vi "NextState.vi"(0 "object in":refnum<class "PrimaryAttackerRole.lvclass">, 2 "Robot in":refnum<class "Robot.lvclass">, 4 "GameRef":refnum<data-value>, 5 "error in (no error)":errorcluster) -> (14 "object out":refnum<class "PrimaryAttackerRole.lvclass">, 16 "Robot out":refnum<class "Robot.lvclass">, 19 "error out":errorcluster)   [LabVIEW 2023, in "PrimaryAttackerRole.lvclass"]
uses:
  PrimaryAttackerRole.lvclass
  C:/Users/ebert/Documents/codes/SSL/repo/SSL_AI/NewSTP/NewRoles/Role_v2_class/Role_v2.lvclass
  Robot_class/Robot.lvclass
  Game_class/Game.lvclass
  PrimaryAttackerRole_states.ctl
  Robot_class/tactics.ctl
  Game_class/Game.lvclass/Game.ctl
  Field_class/Field.lvclass/Field.ctl
  Robot_class/Robot.lvclass/Robot.ctl
  Game_class/Read FieldRef.vi
  Field_class/Read enemyGoalPosition.vi
  Robot_class/Write tactic.vi
  Field_class/Field.lvclass
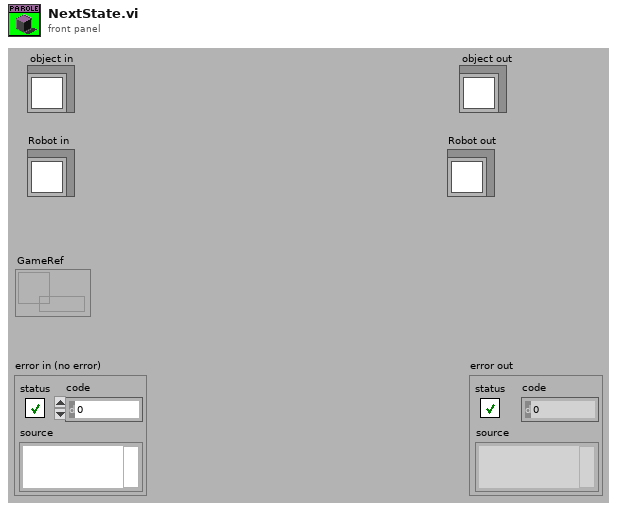
[diagram p1: front panel]
types:
  T1 = typedef "PrimaryAttackerRole.lvclass/PrimaryAttackerRole_states.ctl" = enum16{"Intercept", "PrepareShot", "Shoot", "Pass"}
  T2 = typedef "tactics.ctl" = enum16{"GoToBallPlacementPosition", "PlaceBall", "GoToBallPlacement", "5Robots", "BallPlacementEnemy", "ReceivePassInFuturePoint", "Roller", "PrepareRollToPassRollerGoTo", "PrepareRollToPassReceiverGoTo", "WaitRoll", "PositionToRoll", "PenaltyAttacker", "PassObserver", "PenaltyDefense", "TableReceiverTactic", "Test", "DefendGoal", "Marker", "FollowAttacker", "DefendArea", "Shoot", "AttackerAimGoal", "AttackerBallOutOfField", "AttackerBlock", "AttackerStop", "Duelist", "Halt", "ZigZag", "GoTo", "Timeout", "KickToBestRobot", "KickToPassReceiver", "PositionToReceivePass", "WaitPass", "Position", "Intercept", "PrepareShot", "Pass"}
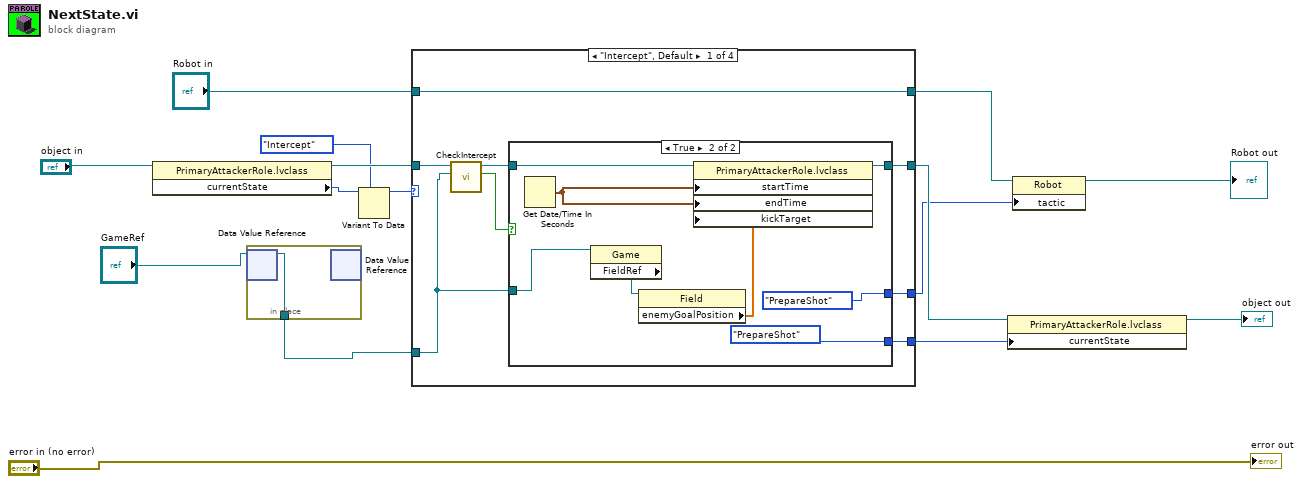
[diagram p0: block diagram]
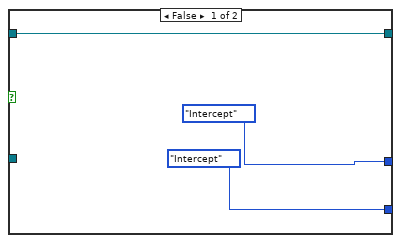
[diagram p2: hidden frame]
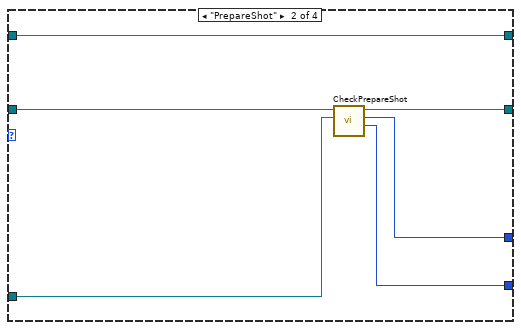
[diagram p3: hidden frame]
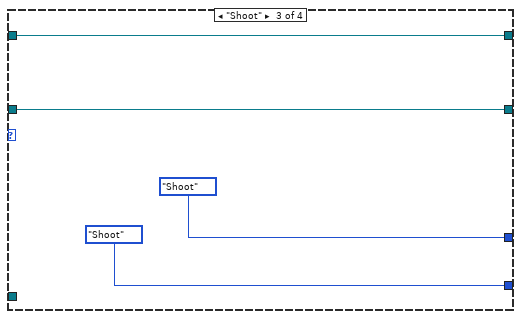
[diagram p4: hidden frame]
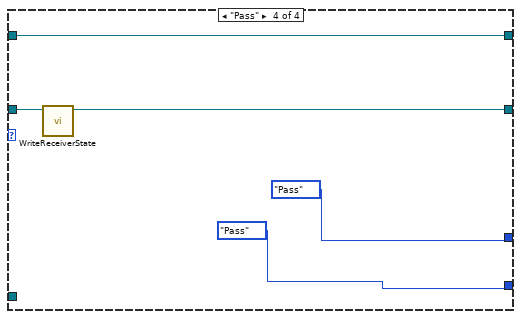
[diagram p5: hidden frame]
diagram:
  n1 = property class="PrimaryAttackerRole.lvclass"(reference="object in") -> (reference out=w13:refnum<class "PrimaryAttackerRole.lvclass">, "currentState"=w7:u8)  [unwired: 1 in, 1 out]
  n2 = in-place {
    in-place-border: [w16] -> w1
    n3 = in-place-dvr #1("GameRef") -> (w16:refnum<class "Game.lvclass">)  [unwired: 1 out]
    n4 = in-place-dvr #1() -> ()  [unwired: 1 in, 2 out]
  }
  n5 = Variant To Data(type=PrimaryAttackerRole_states."Intercept" ("Enum"), Variant=w7) -> (data=w5:T1)  [unwired: 1 in, 1 out]
  n6 = case shown="\"Intercept\", Default" w5 {
    tunnel: [w22 w38 PrimaryAttackerRole_states."Shoot" ("Enum") PrimaryAttackerRole_states."Pass" ("Enum")] -> w3
    tunnel: w1 -> [w17 w37 _ _]
    tunnel: w13 -> [w24 w41 w43 w48]
    tunnel: [w19 w40 w43 w47] -> w14
    tunnel: [w21 w39 tactics."Shoot" ("tactic") tactics."Pass" ("tactic")] -> w4
    tunnel: "Robot in" -> [w18 w36 w42 w46]
    tunnel: [w18 w36 w42 w46] -> w8
    frame "Intercept", Default {
      n7 = call-dynamic "CheckIntercept.vi"("Game"=w17, "object in"=w24) -> ("intercepted"=w23:bool, "object out"=w20:refnum<class "PrimaryAttackerRole.lvclass">)  [unwired: 7 in, 1 out]
      n8 = case shown="True" w23 {
        tunnel: [PrimaryAttackerRole_states."Intercept" ("Enum") PrimaryAttackerRole_states."PrepareShot" ("Enum")] -> w22
        tunnel: [tactics."Intercept" ("tactic") tactics."PrepareShot" ("tactic")] -> w21
        tunnel: w20 -> [w25 w33]
        tunnel: [w25 w32] -> w19
        tunnel: w17 -> [_ w28]
        frame False {
        }
        frame True {
          n9 = Get Date/Time In Seconds() -> (seconds since 1Jan1904=w31:timestamp)
          n10 = property class="Game"(reference=w28) -> ("FieldRef"=w30:refnum<class "Field.lvclass">)  [unwired: 1 in, 2 out]
          n11 = property class="Field"(reference=w30) -> ("enemyGoalPosition"=w29:dbl[])  [unwired: 1 in, 2 out]
          n12 = property class="PrimaryAttackerRole.lvclass"(reference=w33, "startTime"=w31, "endTime"=w31, "kickTarget"=w29) -> (reference out=w32:refnum<class "PrimaryAttackerRole.lvclass">)  [unwired: 1 in, 1 out]
        }
      }
    }
    frame "PrepareShot" {
      n13 = call-dynamic "CheckPrepareShot.vi"("Game"=w37, "object in"=w41) -> ("nextState"=w38:T1, "tactic"=w39:T2, "object out"=w40:refnum<class "PrimaryAttackerRole.lvclass">)  [unwired: 6 in, 1 out]
    }
    frame "Shoot" {
    }
    frame "Pass" {
      n14 = call-dynamic "WriteReceiverState.vi"("PrimaryAttackerRole in"=w48) -> ("PrimaryAttackerRole out"=w47:refnum<class "PrimaryAttackerRole.lvclass">)  [unwired: 9 in, 1 out]
    }
  }
  n15 = property class="PrimaryAttackerRole.lvclass"(reference=w14, "currentState"=w3) -> (reference out=→"object out":refnum<class "PrimaryAttackerRole.lvclass">)  [unwired: 1 in, 1 out]
  n16 = property class="Robot"(reference=w8, "tactic"=w4) -> (reference out=→"Robot out":refnum<class "Robot.lvclass">)  [unwired: 1 in, 1 out]
  "error out" <- "error in (no error)"
